vi "Set Constants.vi"(8 "error in":errorcluster) -> (0 "error out":errorcluster)   [LabVIEW 2015]
uses:
  <vilib>/Utility/config.llb/Read Key (String).vi
  Constants.vi
  <vilib>/Utility/config.llb/NI_LVConfig.lvlib
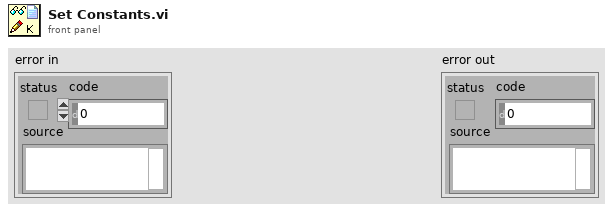
[diagram p1: front panel]
types:
  T1 = cluster{"proportional gain (Kc)":dbl, "integral time (Ti, min)":dbl, "derivative time (Td, min)":dbl}
  T2 = typedef "NI_LVConfig.lvlib/Config Data RefNum.ctl" = refnum<k1>
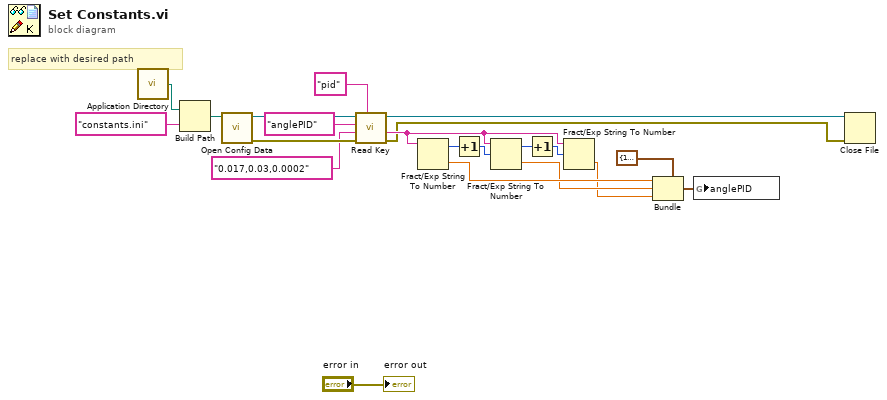
[diagram p0: block diagram]
diagram:
  # "replace with desired path"
  n1 = call <vilib>:"Application Directory.vi"() -> ("Application Directory"=w1:path)
  n2 = Build Path(base path=w1, name or relative path="constants.ini") -> (appended path=w20:path)
  n3 = call <vilib>:"Open Config Data.vi"("configuration file path"=w20) -> ("error out"=w17:errorcluster, "refnum"=w16:T2)  [unwired: 8 in, 1 out]
  n4 = call-poly <vilib>:"Read Key.vi"("section"="pid", "error in (no error)"=w17, "default value"="0.017,0.03,0.0002" ("value"), "key"="anglePID", "refnum"=w16) -> ("error out"=w2:errorcluster, "value"=w9:string, "refnum out"=w3:T2)  [unwired: 3 in, 1 out]
  n5 = Fract/Exp String To Number(string=w9) -> (offset past number=w13:i32, number=w8:dbl)  [unwired: 3 in]
  n6 = Increment(x=w13) -> (x+1=w12:i32)
  n7 = Fract/Exp String To Number(string=w9, offset=w12) -> (offset past number=w11:i32, number=w7:dbl)  [unwired: 2 in]
  n8 = Increment(x=w11) -> (x+1=w10:i32)
  n9 = Fract/Exp String To Number(string=w9, offset=w10) -> (number=w6:dbl)  [unwired: 2 in, 1 out]
  n10 = Bundle(cluster=T1 {"proportional gain (Kc)"=1.0, "integral time (Ti, min)"=0.01, "derivative time (Td, min)"=0.0} ("PID gains"), "proportional gain (Kc)"=w8, "integral time (Ti, min)"=w7, "derivative time (Td, min)"=w6) -> (w4:T1)
  n11 = global write "Constants.vi" "anglePID"(w4) -> ()
  n12 = Close File(refnum=w3, error in=w2) -> ()  [unwired: 2 out]
  "error out" <- "error in"
